vi "AlliGator Define ROI Selection Criteria.vi"(8 "Error In":errorcluster) -> (0 "Error Out":errorcluster, 1 "ROI Characteristics Selection":T1, 2 "ROI Characteristics Min out":T2, 3 "ROI Characteristics Max out":T2)   [LabVIEW 2021, in "AlliGator Source Image.lvlib"]
doc: "Dialog to define selection/rejection criteria for ROIs based on computed characteristics."
uses:
  AlliGator Source Image.lvlib
  Image/Image ROI Statistics.ctl
  Image/Image.lvlib
panel:
  out "Cancelled?":bool
  in  "Cancel":bool
  in  "OK":bool
  in  "ROI Characteristics Max":T2 caption="Max"
  in  "ROI Characteristics Min":T2
  in  "ROI Characteristics Selection":T1
  # "Define min and max allowable values for each selected criterion.\nROIs not verifying these conditions will be deleted."
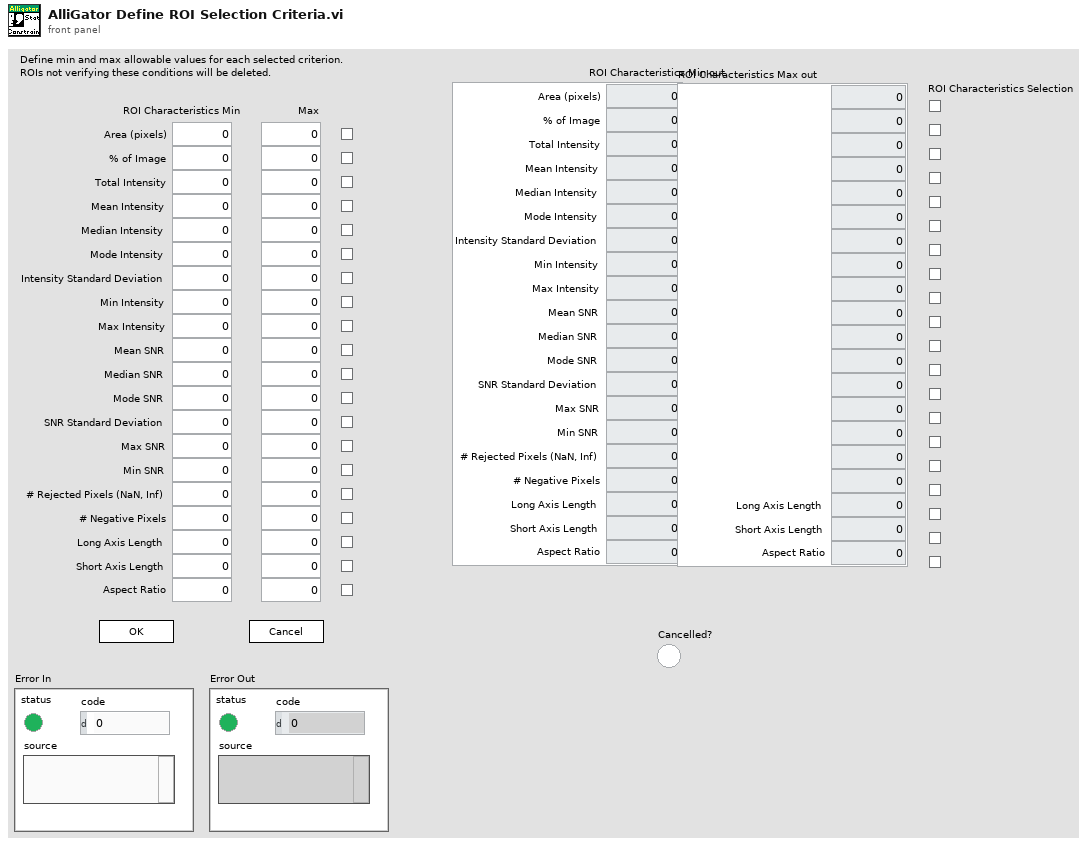
[diagram p1: front panel]
types:
  T1 = cluster{"Area (pixels)":bool, "% of Image":bool, "Total Intensity":bool, "Mean Intensity":bool, "Median Intensity":bool, "Mode Intensity":bool, "Intensity Standard Deviation":bool, "Min Intensity":bool, "Max Intensity":bool, "Mean SNR":bool, "Median SNR":bool, "Mode SNR":bool, "SNR Standard Deviation":bool, "Max SNR":bool, "Min SNR":bool, "# Rejected Pixels (NaN, Inf)":bool, "# Negative Pixels":bool, "Long Axis Length":bool, "Short Axis Length":bool, "Aspect Ratio":bool}
  T2 = typedef "Image.lvlib/Image ROI Statistics.ctl" = cluster{"Area (pixels)":dbl, "% of Image":dbl, "Total Intensity":dbl, "Mean Intensity":dbl, "Median Intensity":dbl, "Mode Intensity":dbl, "Intensity Standard Deviation":dbl, "Min Intensity":dbl, "Max Intensity":dbl, "Mean SNR":dbl, "Median SNR":dbl, "Mode SNR":dbl, "SNR Standard Deviation":dbl, "Max SNR":dbl, "Min SNR":dbl, "# Rejected Pixels (NaN, Inf)":dbl, "# Negative Pixels":dbl, "Long Axis Length":dbl, "Short Axis Length":dbl, "Aspect Ratio":dbl}
  T3 = enum32{"Invalid", "Standard", "Closed", "Hidden", "Minimized", "Maximized"}
  T4 = cluster{"[0]":dbl, "[1]":dbl, "[2]":dbl, "[3]":dbl, "[4]":dbl, "[5]":dbl, "[6]":dbl, "[7]":dbl, "[8]":dbl, "[9]":dbl, "[10]":dbl, "[11]":dbl, "[12]":dbl, "[13]":dbl, "[14]":dbl, "[15]":dbl, "[16]":dbl, "[17]":dbl, "[18]":dbl, "[19]":dbl}
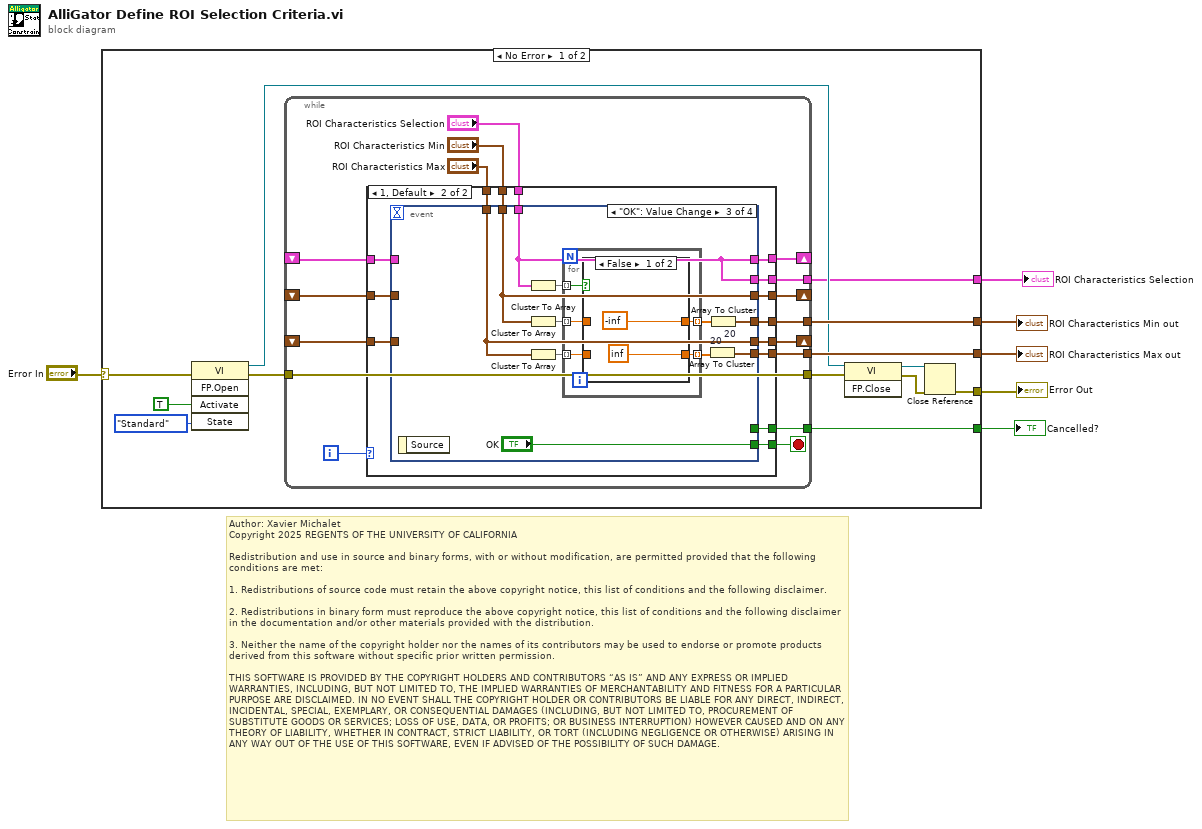
[diagram p0: block diagram]
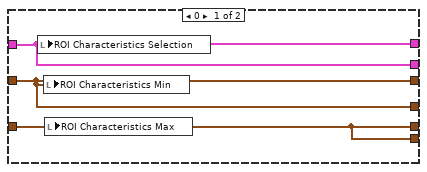
[diagram p2: hidden frame]
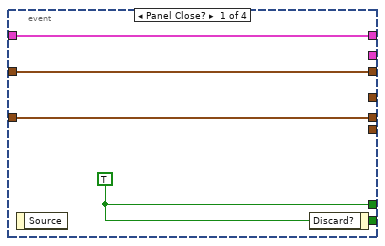
[diagram p3: hidden frame]
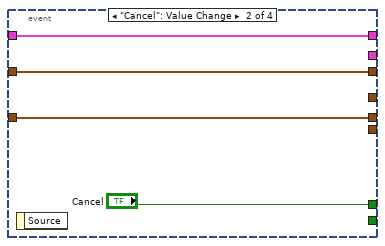
[diagram p4: hidden frame]
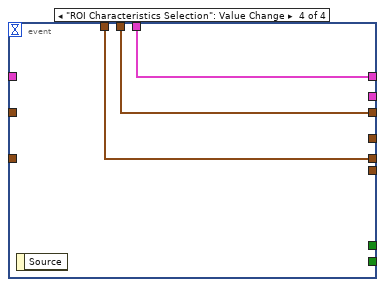
[diagram p6: hidden frame]
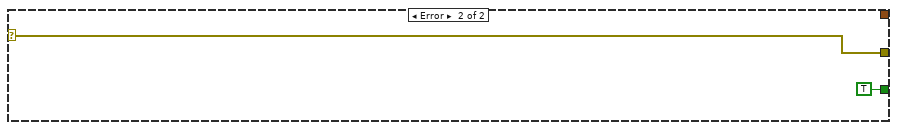
[diagram p7: hidden frame]
diagram:
  # "Author: Xavier Michalet\nCopyright 2025 REGENTS OF THE UNIVERSITY OF CALIFORNIA\n\nRedistribution and use in source and binary forms, with or without modification, are permitted provided that the following conditions are met:\n\n1. Redistributions of source code must retain the above copyright notice, this list of conditions and the following disclaimer.\n\n2. Redistributions in binary form must reproduce the above copyright notice, this list of conditions and the following disclaimer in the documentation and/or other materials provided with the distribution.\n\n3. Neither the name of the copyright holder nor the names of its contributors may be used to endorse or promote products derived from this software without specific prior written permission.\n\nTHIS SOFTWARE IS PROVIDED BY THE COPYRIGHT HOLDERS AND CONTRIBUTORS “AS IS” AND ANY EXPRESS OR IMPLIED WARRANTIES, INCLUDING, BUT NOT LIMITED TO, THE IMPLIED WARRANTIES OF MERCHANTABILITY AND FITNESS FOR A PARTICULAR PURPOSE ARE DISCLAIMED. IN NO EVENT SHALL THE COPYRIGHT HOLDER OR CONTRIBUTORS BE LIABLE FOR ANY DIRECT, INDIRECT, INCIDENTAL, SPECIAL, EXEMPLARY, OR CONSEQUENTIAL DAMAGES (INCLUDING, BUT NOT LIMITED TO, PROCUREMENT OF SUBSTITUTE GOODS OR SERVICES; LOSS OF USE, DATA, OR PROFITS; OR BUSINESS INTERRUPTION) HOWEVER CAUSED AND ON ANY THEORY OF LIABILITY, WHETHER IN CONTRACT, STRICT LIABILITY, OR TORT (INCLUDING NEGLIGENCE OR OTHERWISE) ARISING IN ANY WAY OUT OF THE USE OF THIS SOFTWARE, EVEN IF ADVISED OF THE POSSIBILITY OF SUCH DAMAGE."
  n1 = case shown="No Error" "Error In" {
    selector: "Error In" -> [w11 w85]
    tunnel: [w16 _] -> w6
    tunnel: [w15 _] -> w5
    tunnel: [w12 TRUE ("Cancel")] -> w4
    tunnel: [w10 w85] -> w2
    tunnel: [w7 _] -> w1
    frame No Error {
      n2 = invoke class="VI" method="FP.Open"(error in=w11, "Activate"=TRUE ("Activate?"), "State"=T3."Standard") -> (reference out=w14:refnum<vi>, error out=w9:errorcluster)  [unwired: 2 in, 3 out]
      n3 = while {
        shift-right: [w34] -> _
        shift-left: _ -> [w33]
        shift-right: [w31] -> _
        shift-left: _ -> [w32]
        shift-right: [w29] -> _
        shift-left: _ -> [w30]
        tunnel: [w24] -> w12
        tunnel: [w23] -> w15
        tunnel: [w22] -> w16
        tunnel: w9 -> [w21]
        tunnel: [w21] -> w8
        tunnel: [w20] -> w7
        i -> [w35]
        stop <- w28 stop-if-true
        n4 = case shown="1, Default" w35 {
          tunnel: [w36 w50] -> w34
          tunnel: w33 -> [w36 w51]
          tunnel: w32 -> [w38 w49]
          tunnel: [w38 w48] -> w31
          tunnel: w30 -> [w37 w47]
          tunnel: [w37 w46] -> w29
          tunnel: [_ w52] -> w28
          tunnel: "ROI Characteristics Selection" -> [_ w45]
          tunnel: "ROI Characteristics Min" -> [_ w44]
          tunnel: "ROI Characteristics Max" -> [_ w43]
          tunnel: [_ w42] -> w24
          tunnel: [w38 w41] -> w23
          tunnel: [w37 w40] -> w22
          tunnel: [w36 w39] -> w20
          frame 0 {
            n5 = local write "ROI Characteristics Selection"(w36) -> ()
            n6 = local write "ROI Characteristics Min"(w38) -> ()
            n7 = local write "ROI Characteristics Max"(w37) -> ()
          }
          frame 1, Default {
            n8 = event shown="[2] \"OK\": Value Change" {
              selector: _ -> [_ _ _ _]
              dyn-events: _ -> [_ _ _ _]
              timeout: _ -> [_ _ _ _]
              tunnel: [w53 _ "OK" _] -> w52
              tunnel: w51 -> [w56 w60 _ _]
              tunnel: [w56 w60 w61 w83] -> w50
              tunnel: w49 -> [w55 w59 _ _]
              tunnel: [w55 w59 w70 w82] -> w48
              tunnel: w47 -> [w54 w58 _ _]
              tunnel: [w54 w58 w69 w81] -> w46
              tunnel: w45 -> [_ _ w61 w83]
              tunnel: w44 -> [_ _ w70 w82]
              tunnel: w43 -> [_ _ w69 w81]
              tunnel: [w53 "Cancel" _ _] -> w42
              tunnel: [_ _ w68 _] -> w41
              tunnel: [_ _ w67 _] -> w40
              tunnel: [_ _ w61 _] -> w39
              event Panel Close? {
                w53 = TRUE ("Discard?")
                n9 = event-data() -> ()  [unwired: 1 in, 1 out]
                n10 = event-data("Discard?"=w53) -> ()  [unwired: 1 in, 1 out]
              }
              event "Cancel": Value Change {
                n11 = event-data() -> ()  [unwired: 1 in, 1 out]
              }
              event "OK": Value Change {
                n12 = event-data() -> ()  [unwired: 1 in, 1 out]
                n13 = Cluster To Array(cluster=w61) -> (array=w66:bool[])
                n14 = Cluster To Array(cluster=w70) -> (array=w65:dbl[])
                n15 = Cluster To Array(cluster=w69) -> (array=w64:dbl[])
                n16 = for {
                  tunnel: w66 -> [w76] mode=indexing
                  tunnel: w65 -> [w75] mode=indexing
                  tunnel: w64 -> [w73] mode=indexing
                  tunnel: [w74] -> w63 mode=indexing
                  tunnel: [w72] -> w62 mode=indexing
                  n17 = case shown="False" w76 {
                    tunnel: w75 -> [_ w80]
                    tunnel: [-inf ("Area (pixels)") w80] -> w74
                    tunnel: w73 -> [_ w79]
                    tunnel: [inf ("Area (pixels)") w79] -> w72
                    frame False {
                    }
                    frame True {
                    }
                  }
                }
                n18 = Array To Cluster "20"(array=w62) -> (cluster=w67:T4)
                n19 = Array To Cluster "20"(array=w63) -> (cluster=w68:T4)
              }
              event "ROI Characteristics Selection": Value Change {
                n20 = event-data() -> ()  [unwired: 1 in, 1 out]
              }
            }
          }
        }
      }
      n21 = invoke class="VI" method="FP.Close"(reference=w14, error in=w8) -> (reference out=w17:refnum<vi>, error out=w18:errorcluster)  [unwired: 1 in, 1 out]
      n22 = Close Reference(reference=w17, error in (no error)=w18) -> (error out=w10:errorcluster)
    }
    frame Error {
    }
  }
  "ROI Characteristics Min out" <- w5
  "ROI Characteristics Max out" <- w6
  "Cancelled?" <- w4
  "Error Out" <- w2
  "ROI Characteristics Selection" <- w1
